vi "getParameters.vi"(11 "LowerM1M3Command in":refnum<class "LowerM1M3Command.lvclass">) -> (2 "Parameters":T1, 3 "LowerM1M3Command out":refnum<class "LowerM1M3Command.lvclass">)   [LabVIEW 2016, in "LowerM1M3Command.lvclass"]
uses:
  LowerM1M3Command.lvclass
  DataTypes/Topics/CommandLowerM1M3.ctl
  DataTypes/Topics/Parts/CommandId.ctl
  LowerM1M3Command.lvclass/LowerM1M3Command.ctl
  DataTypes/Topics/M1M3SupportTopics.lvlib
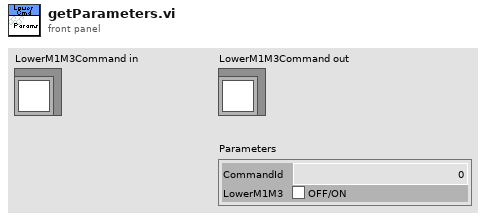
[diagram p1: front panel]
types:
  T1 = typedef "M1M3SupportTopics.lvlib/CommandLowerM1M3.ctl" = cluster{"CommandId":T2, "LowerM1M3":bool}
  T2 = typedef "M1M3SupportTopics.lvlib/CommandId.ctl" = i32
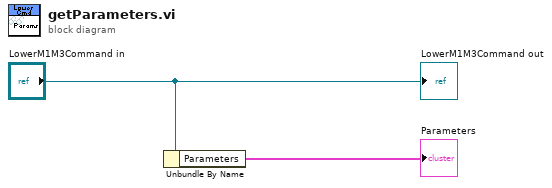
[diagram p0: block diagram]
diagram:
  n1 = Unbundle By Name("LowerM1M3Command in") -> ("Parameters"=→"Parameters":T1)
  "LowerM1M3Command out" <- "LowerM1M3Command in"
